vi "QIcon.vi"(8 "Error In":errorcluster, 10 "fileName":string) -> (0 "Error Out":errorcluster, 3 "New QIcon":refnum<class "QIcon.lvclass">)   [LabVIEW 2014, in "QIcon.lvclass"]
doc: "LabVIEW-specific documentation is not yet available. See <b>https://doc.qt.io/qt-5/qicon.html#QIcon</b>"
uses:
  QIcon.lvclass
  LQ Core/LQSerialData/LQSerialData.lvclass/LQSerialData.ctl
  LQ Core/LQ Core.lvlib
  LQ Core/LQSerialData/LQSerialData.lvclass
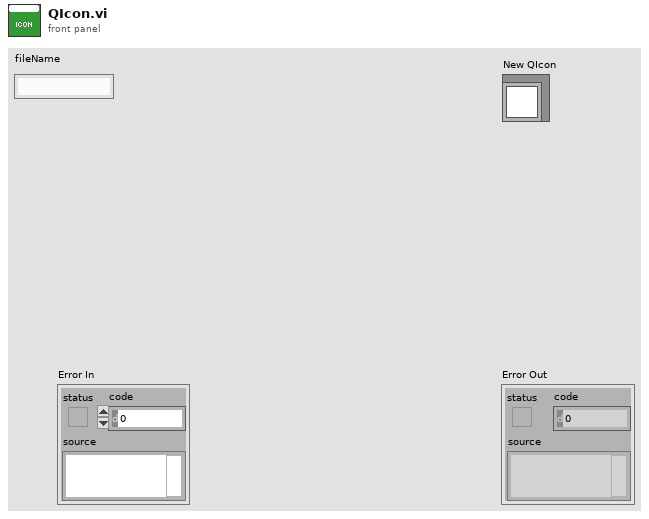
[diagram p1: front panel]
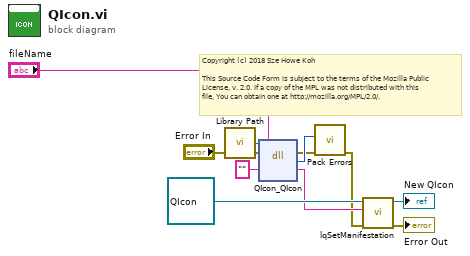
[diagram p0: block diagram]
diagram:
  # "Copyright (c) 2018 Sze Howe Koh\n\nThis Source Code Form is subject to the terms of the Mozilla Public\nLicense, v. 2.0. If a copy of the MPL was not distributed with this\nfile, You can obtain one at http://mozilla.org/MPL/2.0/."
  n1 = call "Library Path.vi"() -> ("Library Path"=w6:path)
  n2 = dll-call lib="?" fn="QIcon_QIcon"(path in=w6, error in="Error In", "_retVal"="", "fileName"="fileName") -> (error out=w4:errorcluster, w5:i32, "_retVal"=w7:string)  [unwired: 2 in, 1 out]
  n3 = call "Pack Errors.vi"("Error In"=w4, "Error Code"=w5) -> ("Error Out"=w3:errorcluster)  [unwired: 9 in]
  n4 = call "lqSetManifestation.vi"("Error In"=w3, "Manifestation"=w7, "LQSerialData in"=refnum<class "QIcon.lvclass"> refnum ("QIcon")) -> ("Error Out"=→"Error Out":errorcluster, "LQSerialData out"=→"New QIcon":refnum<class "QIcon.lvclass">)  [unwired: 7 in]
